vi "Temperature.vi"() -> ()   [LabVIEW 2017]
panel:
  out "Thermometer":dbl(slide) scale=0.0..100.0
  in  "Temperature (F)":dbl(slide) scale=0.0..200.0
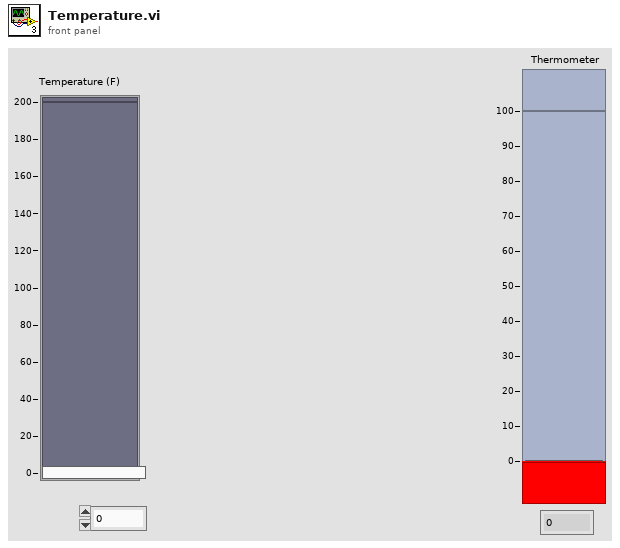
[diagram p1: front panel]
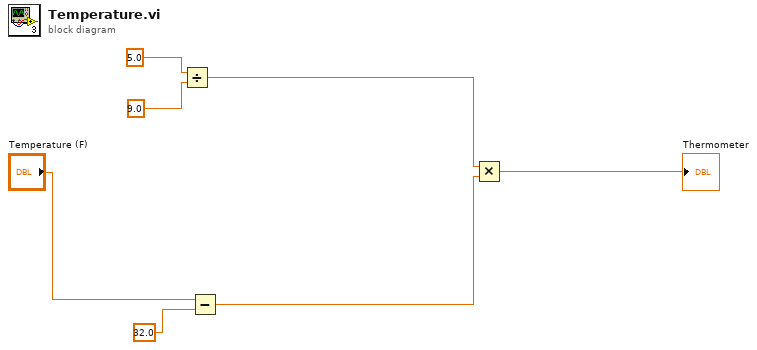
[diagram p0: block diagram]
diagram:
  n1 = Divide(x=5.0 ("y"), y=9.0 ("x/y")) -> (x/y=w3:dbl)
  n2 = Subtract(x="Temperature (F)", y=32.0 ("x")) -> (x-y=w2:dbl)
  n3 = Multiply(x=w3, y=w2) -> (x*y=→"Thermometer":dbl)
